vi "TCP Server Module(Multi-Loop Support).vi"(7 "Name (\"\" to Use UUID)":string="Event CSM Tiny") -> ()   [LabVIEW 2017, in "Multi-Loop Module Example.lvlib"]
doc: "------------- lvcsm -------------\n[CSMStates]\nItem 0 = \"Event Structure\"\nItem 1 = \"Idle\"\nItem 2 = \"CSM Documentation\"\nItem 3 = \"VI Reference\"\nItem 4 = \"Error Handler\"\nItem 5 = \"Critical Error\"\nItem 6 = \"Target Error\"\nItem 7 = \"Target Timeout Error\"\nItem 8 = \"Async Response\"\nItem 9 = \"Response\"\nItem 10 = \"Async Message Posted\"\nItem 11 = \"Initialize Core Data\"\nItem 12 = \"Exit\"\nItem 13 = \"Data: Initialize\"\nItem 14 = \"Data: Cleanup\"\nItem 15 = \"Events: Register\"\nItem 16 = \"Events: Unregister\"\nItem 17 = \"UI: Initialize\"\nItem 18 = \"UI: Cursor Set\"\nItem 19 = \"UI: Front Panel State\"\nItem 20 = \"Macro: Initialize\"\nItem 21 = \"Macro: Exit\"\nItem 22 = \"TCP: Send\"\nItem 23 = \"TCP: Receive\"\n\n[CSMStatus]\nItem 0 = \"Error Occurred@Error Handler\"\nItem 1 = \"TCP Received@TCP: Receive\"\nItem 2 = \"TCP Disconnected@\"\nItem 3 = \"TCP Connected@\""
uses:
  Multi-Loop Module Example.lvlib
  user.lib/_NEVSTOP/Communicable State Machine(CSM)/AdvanceAPI/CSM - Make String Arguments Safe.vi
  user.lib/_NEVSTOP/Communicable State Machine(CSM)/AdvanceAPI/CSM - Break Down Multiple States String.vi
  user.lib/_NEVSTOP/Communicable State Machine(CSM)/AdvanceAPI/CSM - Compact Multiple States.vi
  user.lib/_NEVSTOP/Communicable State Machine(CSM)/AdvanceAPI/CSM - Keywords.vi
  user.lib/_NEVSTOP/Communicable State Machine(CSM)/AdvanceAPI/CSM - List Modules.vi
  user.lib/_NEVSTOP/Communicable State Machine(CSM)/Communicable State Machine.lvlib
panel:
  in  "Send String":string
  out "Connected":bool
  out "TCP Received":string
  out "TCP":refnum<k5>
  out "State History":string
  # "#CSM-Example Overview"
  # "#CSM-Example Instructions"
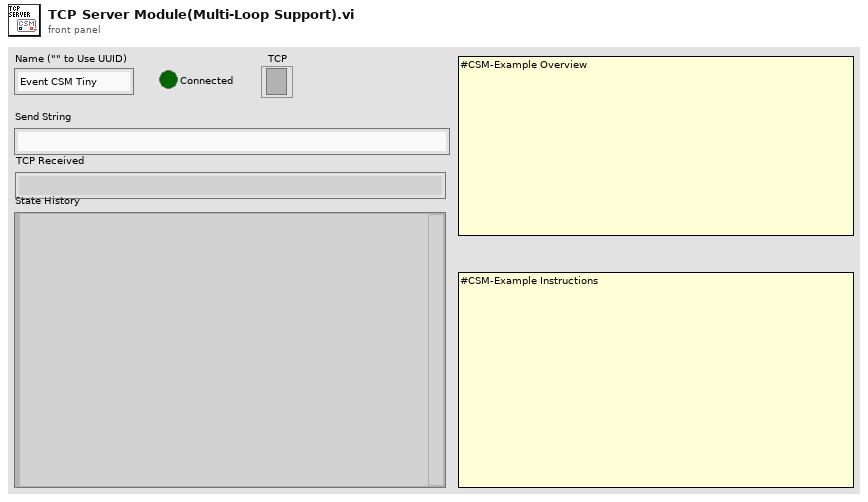
[diagram p1: front panel]
types:
  T1 = enum32{"Invalid", "Standard", "Closed", "Hidden", "Minimized", "Maximized"}
  T2 = enum32{"invalid app kind", "Development System", "Run Time System", "Student Edition", "Embedded LabVIEW", "Evaluation", "Custom"}
  T3 = typedef "Communicable State Machine.lvlib/_CSM_Response Source Message.ctl" = cluster{"‘State":string, "’Arguments":string, "’Error":errorcluster}
  T4 = cluster{"Current VI Reference":refnum<vi>, "Close Panel on Exit?":bool}
  T5 = cluster{"Core":cluster{"Current VI Reference":refnum<vi>, "Close Panel on Exit?":bool}, "Your Boolean data":bool, "Your string data":string}
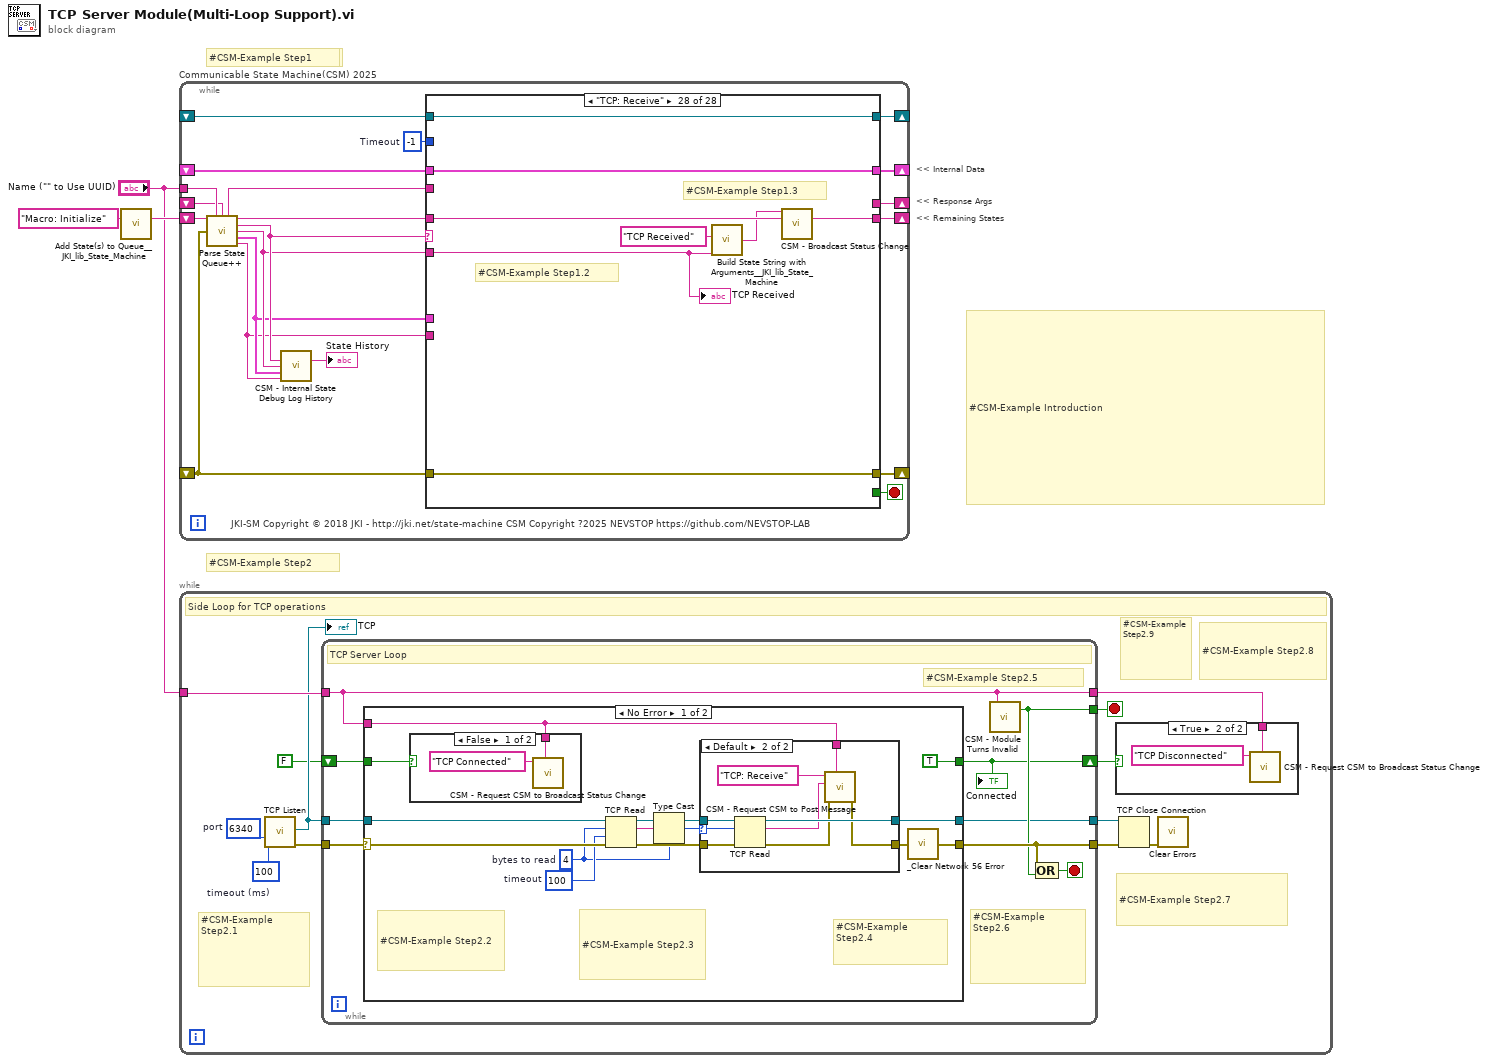
[diagram p0: block diagram]
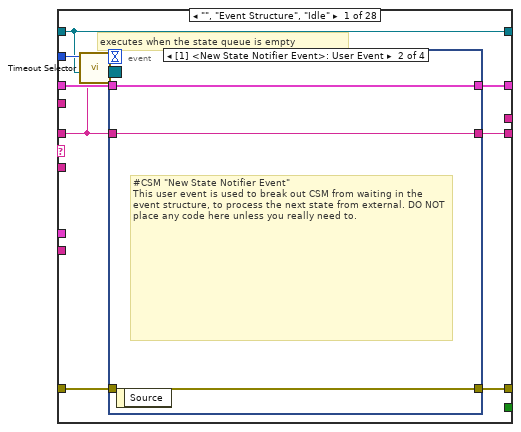
[diagram p2: hidden frame]
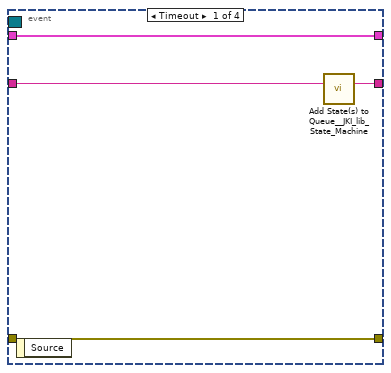
[diagram p3: hidden frame]
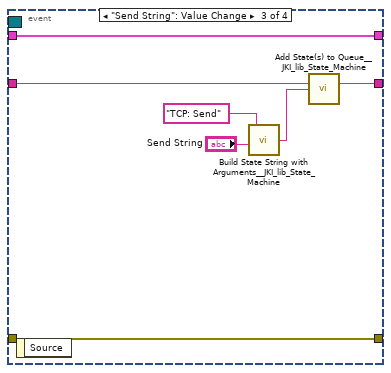
[diagram p4: hidden frame]
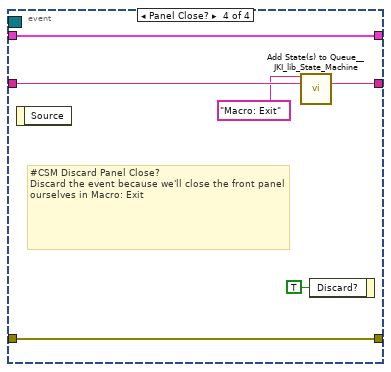
[diagram p5: hidden frame]
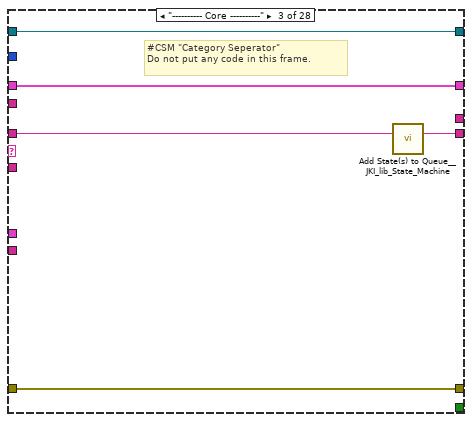
[diagram p7: hidden frame]
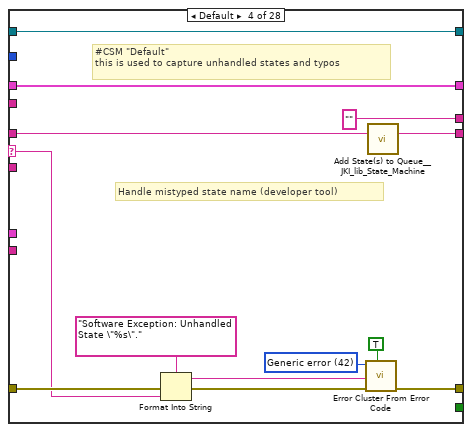
[diagram p8: hidden frame]
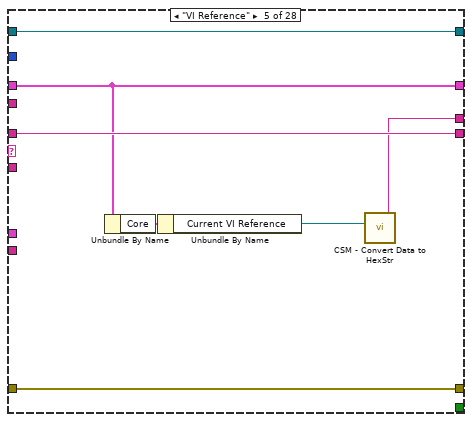
[diagram p9: hidden frame]
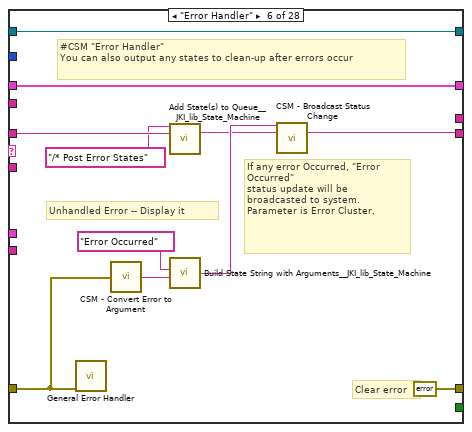
[diagram p10: hidden frame]
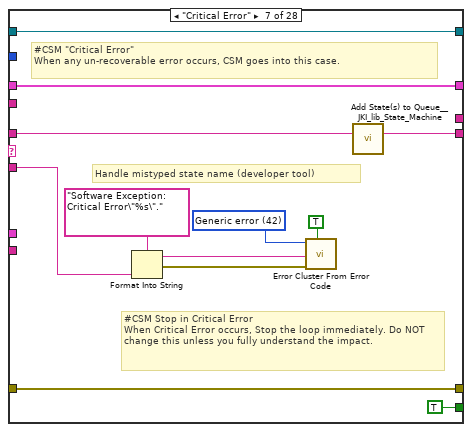
[diagram p11: hidden frame]
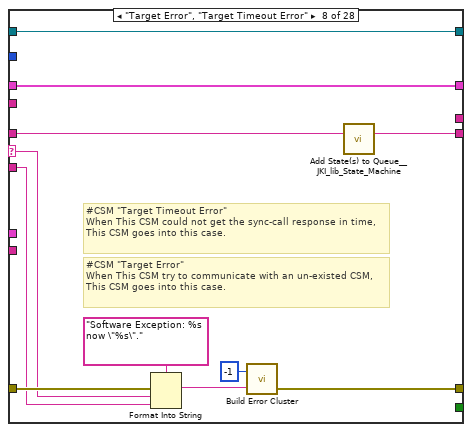
[diagram p12: hidden frame]
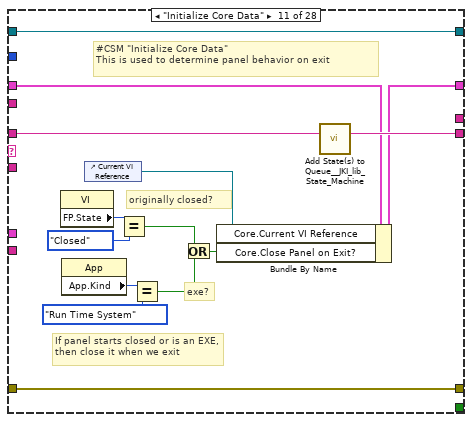
[diagram p15: hidden frame]
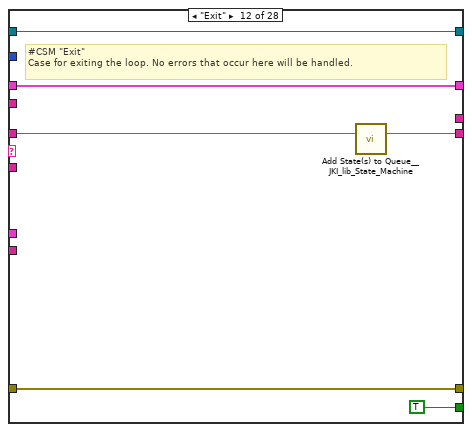
[diagram p16: hidden frame]
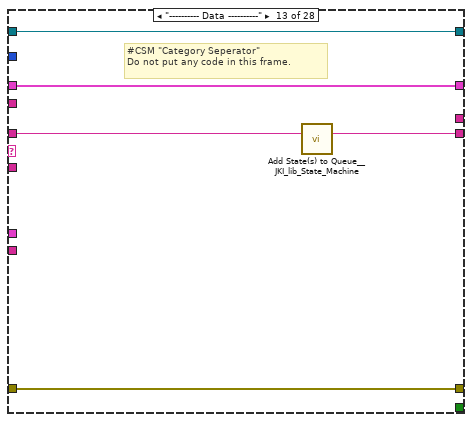
[diagram p17: hidden frame]
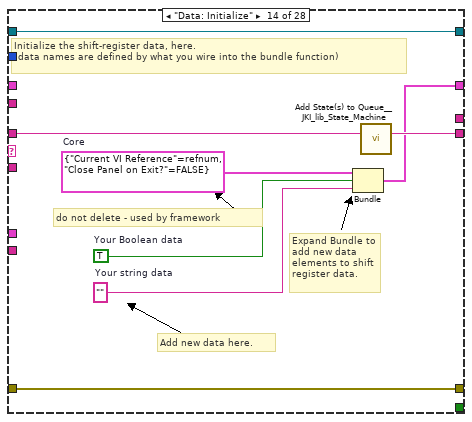
[diagram p18: hidden frame]
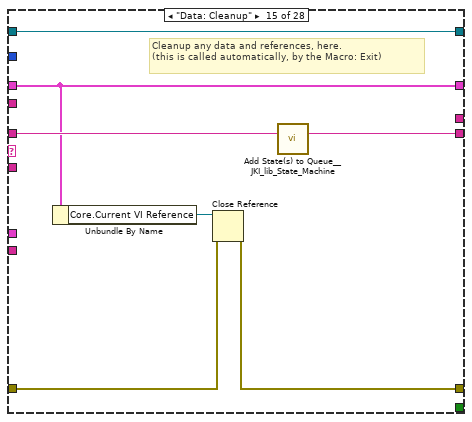
[diagram p19: hidden frame]
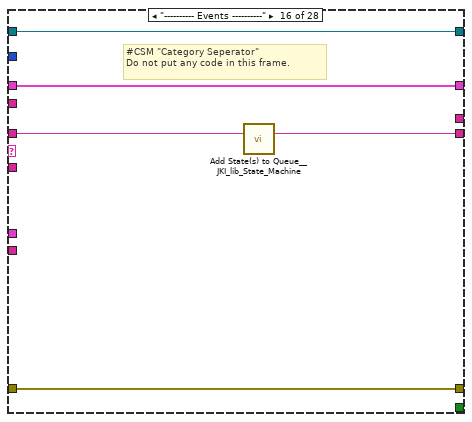
[diagram p20: hidden frame]
diagram:
  # "#CSM-Example Step1"
  # "#CSM-Example Step2"
  # "#CSM-Example Step1"
  # "#CSM-Example Introduction"
  # "<< Internal Data"
  # "<< Response Args"
  # "<< Remaining States"
  n1 = call <vilib>:"Add State(s) to Queue__JKI_lib_State_Machine.vi"("State(s) in (\"\")"="Macro: Initialize") -> ("States Out"=w2:string)  [unwired: 14 in]
  n2 = while "Communicable State Machine(CSM) 2025" {
    shift-right: [w18] -> _
    shift-left: _ -> [w17]
    shift-right: [w21] -> _
    shift-left: _ -> [w15]
    shift-right: [w20] -> _
    shift-left: w2 -> [w22]
    tunnel: "Name (\"\" to Use UUID)" -> [w11]
    shift-right: [w14] -> _
    shift-left: _ -> [w5]
    shift-right: [w13] -> _
    shift-left: _ -> [w12]
    stop <- w19 stop-if-true
    w16 = -1  # Timeout
    # "JKI-SM Copyright © 2018 JKI - http://jki.net/state-machine CSM Copyright ?2025 NEVSTOP https://github.com/NEVSTOP-LAB"
    n3 = call "Parse State Queue++.vi"("State Queue"=w22, "Name (\"\" to Use UUID)"=w11, "Response Arguments"=w5, "Previous Error"=w15) -> ("Name Used"=w6:string, "Remaining States"=w23:string, "Current State"=w10:string, "Arguments"=w9:string, "Additional Information"=w8:T3, "Source CSM"=w7:string)  [unwired: 6 in]
    n4 = call "CSM - Internal State Debug Log History.vi"("State"=w10, "Arguments (\"\")"=w9, ">> Response Source Message >>"=w8, "Source (\"\")"=w7) -> ("Debug Log"=→"State History":string)  [unwired: 11 in]
    n5 = case shown="\"TCP: Receive\"" w10 {
      selector: w10 -> [_ _ _ w64 _ _ _ w108 _ _ _ _ _ _ _ _ _ _ _ _ _ _ _ _ _ _ _ _]
      tunnel: w23 -> [w24 w55 w61 w68 w80 w92 w102 w110 w118 w122 w137 w143 w148 w156 w163 w168 w175 w179 w185 w190 w197 w213 w283 w289 w300 w303 w314 w321]
      tunnel: w9 -> [_ _ _ _ _ _ w95 w109 _ _ _ _ _ _ _ _ _ _ _ _ w192 w207 _ _ _ _ w305 w316]
      tunnel: w17 -> [w31 w54 w58 w66 w79 w90 w103 w112 w117 w121 w130 w141 w145 _ w158 w165 w174 w178 w182 w188 w195 w209 w280 w286 w297 w302 w313 w320]
      tunnel: [w30 w56 w59 w70 w81 errorcluster {"status"=FALSE, "code"=0, "source"=""} ("error out") w104 w106 w119 w123 w134 w140 w146 w153 w159 w166 w169 w177 w183 w187 w193 w210 w281 w287 w298 w304 w306 w322] -> w21
      tunnel: w15 -> [w29 w56 w59 w69 w81 w82 w104 w114 w119 w123 w134 w140 w146 w153 w160 w166 _ w180 w183 w187 w194 w211 w281 w287 w298 w304 _ w322]
      tunnel: [w32 w55 w60 w67 w80 w83 w101 w113 w118 w122 w136 w142 w147 w155 w162 w167 w175 w179 w184 w189 w196 w212 w282 w288 w299 w303 w314 w318] -> w20
      tunnel: [_ _ _ _ _ _ TRUE _ _ _ _ TRUE _ _ _ _ _ _ _ _ _ _ _ _ _ _ _ _] -> w19
      tunnel: [w28 w54 w58 w66 w79 w90 w103 w112 w117 w121 w135 w141 w145 w154 w158 w165 w174 w178 w182 w188 w195 w209 w280 w286 w297 w302 w313 w320] -> w18
      tunnel: w16 -> [w27 _ _ _ _ _ _ _ _ _ _ _ _ _ _ _ _ _ _ _ _ _ _ _ _ _ _ _]
      tunnel: w7 -> [_ _ _ _ _ _ _ _ _ _ _ _ _ _ _ _ _ _ _ _ _ _ _ _ _ _ _ _]
      tunnel: w8 -> [_ _ _ _ _ _ _ _ _ _ _ _ _ _ _ _ _ _ _ _ _ _ _ _ _ _ _ _]
      tunnel: [_ _ _ "" w75 _ _ _ _ _ _ _ _ _ _ _ _ _ _ _ _ _ _ _ _ _ _ _] -> w14
      tunnel: [w26 w53 w57 w62 w78 w88 w93 w111 w116 w120 w124 w138 w144 w149 w157 w164 w173 w176 w181 w186 w191 w206 w279 w284 w290 w301 w312 w319] -> w13
      tunnel: w12 -> [w26 w53 w57 w62 w78 w88 w93 w111 w116 w120 w124 w138 w144 w149 w157 w164 _ w176 w181 w186 w191 w206 w279 w284 w290 w301 w312 w319]
      tunnel: w6 -> [_ _ _ _ _ _ _ _ _ _ _ _ _ _ _ _ w172 _ _ _ _ _ _ _ _ _ _ _]
      frame "", "Event Structure", "Idle" {
        # "executes when the state queue is empty"
        n6 = call "Timeout Selector.vi"("Remaining States"=w24, "Timeout Expected"=w27) -> ("Timeout"=w25:i32)  [unwired: 5 in]
        n7 = event shown="[1] <New State Notifier Event>: User Event" {
          selector: w26 -> [_ _ _ _]
          dyn-events: _ -> [_ _ _ _]
          timeout: w25 -> [_ _ _ _]
          tunnel: w24 -> [w36 w38 w44 w52]
          tunnel: [w35 w38 w43 w51] -> w32
          tunnel: w31 -> [w33 w39 w45 w49]
          tunnel: [w34 w37 w46 w50] -> w30
          tunnel: w29 -> [w34 w37 w46 w50]
          tunnel: [w33 w39 w45 w49] -> w28
          event Timeout {
            n8 = event-data() -> ()  [unwired: 1 in, 1 out]
            n9 = call <vilib>:"Add State(s) to Queue__JKI_lib_State_Machine.vi"("State(s) in (\"\")"=w36) -> ("States Out"=w35:string)  [unwired: 14 in]
          }
          event User Event {
            # "#CSM \"New State Notifier Event\"\nThis user event is used to break out CSM from waiting in the event structure, to process the next state from external. DO NOT place any code here unless you really need to."
            n10 = event-data() -> ()  [unwired: 1 in, 1 out]
          }
          event "Send String": Value Change {
            n11 = event-data() -> ()  [unwired: 1 in, 1 out]
            n12 = call <vilib>:"Build State String with Arguments__JKI_lib_State_Machine.vi"("Arguments (\"\")"="Send String", "State"="TCP: Send") -> ("State with Arguments"=w41:string)  [unwired: 4 in]
            n13 = call <vilib>:"Add State(s) to Queue__JKI_lib_State_Machine.vi"("State(s) in (\"\")"=w44, "State(s) at Back (\"\")"=w41) -> ("States Out"=w43:string)  [unwired: 13 in]
          }
          event Panel Close? {
            # "#CSM Discard Panel Close?\nDiscard the event because we'll close the front panel ourselves in Macro: Exit"
            n14 = event-data() -> ()  [unwired: 1 in, 1 out]
            n15 = call <vilib>:"Add State(s) to Queue__JKI_lib_State_Machine.vi"("State(s) in Front (\"\")"="Macro: Exit", "State(s) in (\"\")"=w52) -> ("States Out"=w51:string)  [unwired: 13 in]
            n16 = event-data("Discard?"=TRUE) -> ()  [unwired: 1 in, 1 out]
          }
        }
      }
      frame "CSM Documentation" {
        # "#CSM README FIRST\n\nCSM is a LabVIEW application framework that builds upon JKI State Machine (JKISM). It follows the pattern of JKISM and extends the keywords to describe message communication between CSM modules, including concepts such as Sync-Message, Async-Message, Subscription/Unsubscription of status - essential elements for creating reusable code modules. For more information, please visit the CSM wiki: https://github.com/NEVSTOP-LAB/JKI-State-Machine-Plus-Plus/wiki\n\nFor instructions on JKI State Machine, visit: http://jki.net/state-machine/\nFor information about CSM, visit: https://github.com/NEVSTOP-LAB"
        # "#CSM \"Documentation\"\nCase for holding CSM Documenation"
      }
      frame "---------- Core ----------" {
        # "#CSM \"Category Seperator\"\nDo not put any code in this frame."
        n17 = call <vilib>:"Add State(s) to Queue__JKI_lib_State_Machine.vi"("State(s) in (\"\")"=w61) -> ("States Out"=w60:string)  [unwired: 14 in]
      }
      frame Default {
        w73 = 42 items=["No error", "Argument error", "Memory is full", "Out of zone", "End of file", "File already open", "Generic file I/O error", "File not found", "File permission error", "Disk is full", "Duplicate path", "Too many files open", "System feature not enabled", "Resource file not found", "Cannot add resource", "Resource not found", "Image not found", "Image memory error", "Pen does not exist", "Config type invalid", "Config token not found", "Config parse error", "Config memory error", "Bad external code format", "Bad external code offset", "External code not present", "Null window", "Destroy window error", "Null menu", "Print aborted", "Bad print record", "Print driver error", "Windows error during printing", "Memory error during printing", "Print dialog error", "Generic print error", "Invalid device refnum", "Device not found", "Device parameter error", "Device unit error", "Cannot open device", "Device call aborted", "Generic error", "Cancelled by user", "Object ID too low", "Object ID too high", "Object not in heap", "Unknown heap", "Unknown object (invalid DefProc)", "Unknown object (DefProc not in table)", "Message out of range", "Invalid (null) method", "Unknown message", "Manager call not supported", "Bad address", "Network operation in progress", "Network operation timed out", "Connection is busy", "Network attribute not supported", "Network error", "Address in use", "System out of memory", "Connection aborted", "Connection refused", "Not connected", "Already connected", "Connection closed", "Initialization error (interapplication manager)", "Bad occurrence", "Wait on unbound occurrence handler", "Occurrence queue overflow", "Datalog type conflict", "Unused", "Unrecognized type (interapplication manager)", "Memory corrupt", "Failed to make temporary DLL", "Old CIN version", "Drag socket not found", "Failed to load drop-object", "Failed to register OLE object", "Failed to release OLE object", "Format specifier type mismatch", "Unknown format specifier", "Too few format specifiers", "Too many format specifiers", "Scan failed", "Newer CIN version", "Error converting to variant", "Runtime menu error", "Password tampered", "Variant attribute not found", "Incompatible variant data type", "Event data is not available", "Event Store is not present", "Occurrence is not found", "Event Queue is not created", "Event info is not available", "Refnum passed is NULL", "Error retrieving Class GUID", "Error retrieving CoClass GUID", "Error retrieving TypeLib GUID.", "Bad built application magic bytes.", "Specific driver is different from the specific driver associated with the Logical Name.", "There is no session opened to the class driver.", "Max Error", "MAX - Error with config objects", "MAX - Error loading configuration", "MAX - Group not supported"]
        # "#CSM \"Default\"\nthis is used to capture unhandled states and typos"
        # "Handle mistyped state name (developer tool)"
        n18 = Format Into String(format string="Software Exception: Unhandled State \"%s\"." ("message"), error in=w69, w64) -> (resulting string=w72:string, error out=w71:errorcluster)  [unwired: 1 in]
        n19 = call <vilib>:"Error Cluster From Error Code.vi"("show call chain? (False)"=TRUE, "error in (no error)"=w71, "error message (\"\")"=w72, "error code (0)"=w73) -> ("error out"=w70:errorcluster)  [unwired: 5 in]
        n20 = call <vilib>:"Add State(s) to Queue__JKI_lib_State_Machine.vi"("State(s) in (\"\")"=w68) -> ("States Out"=w67:string)  [unwired: 14 in]
      }
      frame "VI Reference" {
        n21 = Unbundle By Name(w79) -> ("Core"=w77:T4)
        n22 = Unbundle By Name(w77) -> ("Current VI Reference"=w76:refnum<vi>)
        n23 = call "CSM - Convert Data to HexStr.vi"("Variant"=w76) -> ("HEX String (0-9,A-F)"=w75:string)  [unwired: 8 in]
      }
      frame "Error Handler" {
        # "#CSM \"Error Handler\"\nYou can also output any states to clean-up after errors occur"
        # "If any error Occurred, \"Error Occurred\" \nstatus update will be broadcasted to system.\nParameter is Error Cluster."
        # "Unhandled Error -- Display it"
        # "Clear error"
        n24 = call <vilib>:"General Error Handler.vi"("error in (no error)"=w82) -> ()  [unwired: 10 in, 5 out]
        n25 = call "CSM - Convert Error to Argument.vi"("Error"=w82) -> ("Argument"=w86:string)  [unwired: 4 in]
        n26 = call <vilib>:"Add State(s) to Queue__JKI_lib_State_Machine.vi"("State(s) in Front (\"\")"="/* Post Error States", "State(s) in (\"\")"=w92) -> ("States Out"=w84:string)  [unwired: 13 in]
        n27 = call <vilib>:"Build State String with Arguments__JKI_lib_State_Machine.vi"("Arguments (\"\")"=w86, "State"="Error Occurred" ("Status with Arguments")) -> ("State with Arguments"=w85:string)  [unwired: 4 in]
        n28 = call "CSM - Broadcast Status Change.vi"("Status With Arguments"=w85, "State Queue"=w84) -> ("Remaining States"=w83:string)  [unwired: 13 in]
      }
      frame "Critical Error" {
        w99 = 42 items=["No error", "Argument error", "Memory is full", "Out of zone", "End of file", "File already open", "Generic file I/O error", "File not found", "File permission error", "Disk is full", "Duplicate path", "Too many files open", "System feature not enabled", "Resource file not found", "Cannot add resource", "Resource not found", "Image not found", "Image memory error", "Pen does not exist", "Config type invalid", "Config token not found", "Config parse error", "Config memory error", "Bad external code format", "Bad external code offset", "External code not present", "Null window", "Destroy window error", "Null menu", "Print aborted", "Bad print record", "Print driver error", "Windows error during printing", "Memory error during printing", "Print dialog error", "Generic print error", "Invalid device refnum", "Device not found", "Device parameter error", "Device unit error", "Cannot open device", "Device call aborted", "Generic error", "Cancelled by user", "Object ID too low", "Object ID too high", "Object not in heap", "Unknown heap", "Unknown object (invalid DefProc)", "Unknown object (DefProc not in table)", "Message out of range", "Invalid (null) method", "Unknown message", "Manager call not supported", "Bad address", "Network operation in progress", "Network operation timed out", "Connection is busy", "Network attribute not supported", "Network error", "Address in use", "System out of memory", "Connection aborted", "Connection refused", "Not connected", "Already connected", "Connection closed", "Initialization error (interapplication manager)", "Bad occurrence", "Wait on unbound occurrence handler", "Occurrence queue overflow", "Datalog type conflict", "Unused", "Unrecognized type (interapplication manager)", "Memory corrupt", "Failed to make temporary DLL", "Old CIN version", "Drag socket not found", "Failed to load drop-object", "Failed to register OLE object", "Failed to release OLE object", "Format specifier type mismatch", "Unknown format specifier", "Too few format specifiers", "Too many format specifiers", "Scan failed", "Newer CIN version", "Error converting to variant", "Runtime menu error", "Password tampered", "Variant attribute not found", "Incompatible variant data type", "Event data is not available", "Event Store is not present", "Occurrence is not found", "Event Queue is not created", "Event info is not available", "Refnum passed is NULL", "Error retrieving Class GUID", "Error retrieving CoClass GUID", "Error retrieving TypeLib GUID.", "Bad built application magic bytes.", "Specific driver is different from the specific driver associated with the Logical Name.", "There is no session opened to the class driver.", "Max Error", "MAX - Error with config objects", "MAX - Error loading configuration", "MAX - Group not supported"]
        # "#CSM Stop in Critical Error\nWhen Critical Error occurs, Stop the loop immediately. Do NOT change this unless you fully understand the impact."
        # "#CSM \"Critical Error\"\nWhen any un-recoverable error occurs, CSM goes into this case."
        # "Handle mistyped state name (developer tool)"
        n29 = Format Into String(format string="Software Exception: Critical Error\"%s\"." ("message"), w95) -> (resulting string=w98:string, error out=w97:errorcluster)  [unwired: 2 in]
        n30 = call <vilib>:"Error Cluster From Error Code.vi"("show call chain? (False)"=TRUE, "error in (no error)"=w97, "error message (\"\")"=w98, "error code (0)"=w99) -> ()  [unwired: 5 in, 1 out]
        n31 = call <vilib>:"Add State(s) to Queue__JKI_lib_State_Machine.vi"("State(s) in (\"\")"=w102) -> ("States Out"=w101:string)  [unwired: 14 in]
      }
      frame "Target Error", "Target Timeout Error" {
        # "#CSM \"Target Error\"\nWhen This CSM try to communicate with an un-existed CSM, This CSM goes into this case."
        # "#CSM \"Target Timeout Error\"\nWhen This CSM could not get the sync-call response in time, This CSM goes into this case."
        n32 = Format Into String(format string="Software Exception: %s now \"%s\"." ("message"), error in=w114, w108, w109) -> (resulting string=w107:string)  [unwired: 1 in, 1 out]
        n33 = call "Build Error Cluster.vi"("String to Prepend to Source (\"\")"=w107, "Code"=-1 ("code")) -> ("error out"=w106:errorcluster)
        n34 = call <vilib>:"Add State(s) to Queue__JKI_lib_State_Machine.vi"("State(s) in (\"\")"=w110) -> ("States Out"=w113:string)  [unwired: 14 in]
      }
      frame "Async Response", "Response" {
        # "#CSM Response Comments\nAfter Message is executed, CSM goes to this state for receive the response.\n    For Async Message(->), \"Async Response\" is used. This CSM will goes to \"Async Message Posted\" immediately and receive the \"Async Response\" after the callee finishes the message.\n    For Sync Message(@),  This CSM will wait until the message is done and immediately goes to \"Response\""
        # "#CSM \"Async Response\"\nHandle Async-call Response (\"Async Response\" for ->)"
        # "#CSM \"Response\"\nHandle Sync-call Response (\"Response\" for -@)"
      }
      frame "Async Message Posted" {
        # "#CSM \"Async Message Posted\"\nAfter Async Message is posted (-> or ->| ), CSM goes to this state for post-action.\nYou can use Argument - State to tell which Async Message is called."
      }
      frame "Initialize Core Data" {
        # "#CSM \"Initialize Core Data\"\nThis is used to determine panel behavior on exit"
        # "originally closed?"
        # "exe?"
        # "If panel starts closed or is an EXE, then close it when we exit"
        n35 = property class="VI"() -> ("FP.State"=w127:T1)  [unwired: 2 in, 2 out]
        n36 = property class="App"() -> ("App.Kind"=w133:T2)  [unwired: 2 in, 2 out]
        n37 = control-ref of="Current VI Reference"() -> (w128:refnum<vi>)
        n38 = Equal?(x=w127, y=T1."Closed" ("Front Panel Window:State")) -> (x = y?=w125:bool)
        n39 = Equal?(x=w133, y=T2."Run Time System" ("Application:Kind")) -> (x = y?=w131:bool)
        n40 = Or(x=w125, y=w131) -> (x .or. y?=w129:bool)
        n41 = Bundle By Name(cluster=w130, "Core.Current VI Reference"=w128, "Core.Close Panel on Exit?"=w129) -> (w135:T5)
        n42 = call <vilib>:"Add State(s) to Queue__JKI_lib_State_Machine.vi"("State(s) in (\"\")"=w137) -> ("States Out"=w136:string)  [unwired: 14 in]
      }
      frame "Exit" {
        # "#CSM \"Exit\"\nCase for exiting the loop. No errors that occur here will be handled."
        n43 = call <vilib>:"Add State(s) to Queue__JKI_lib_State_Machine.vi"("State(s) in (\"\")"=w143) -> ("States Out"=w142:string)  [unwired: 14 in]
      }
      frame "---------- Data ----------" {
        # "#CSM \"Category Seperator\"\nDo not put any code in this frame."
        n44 = call <vilib>:"Add State(s) to Queue__JKI_lib_State_Machine.vi"("State(s) in (\"\")"=w148) -> ("States Out"=w147:string)  [unwired: 14 in]
      }
      frame "Data: Initialize" {
        w150 = T4 {"Current VI Reference"=refnum, "Close Panel on Exit?"=FALSE}  # Core
        w152 = TRUE  # Your Boolean data
        w151 = ""  # Your string data
        # "do not delete - used by framework"
        # "Expand Bundle to add new data elements to shift register data."
        # "Add new data here."
        # "Initialize the shift-register data, here.\n(data names are defined by what you wire into the bundle function)"
        n45 = Bundle("Core"=w150, "Your Boolean data"=w152, "Your string data"=w151) -> (w154:T5)  [unwired: 1 in]
        n46 = call <vilib>:"Add State(s) to Queue__JKI_lib_State_Machine.vi"("State(s) in (\"\")"=w156) -> ("States Out"=w155:string)  [unwired: 14 in]
      }
      frame "Data: Cleanup" {
        # "Cleanup any data and references, here.\n(this is called automatically, by the Macro: Exit)"
        n47 = Unbundle By Name(w158) -> ("Core.Current VI Reference"=w161:refnum<vi>)
        n48 = Close Reference(reference=w161, error in (no error)=w160) -> (error out=w159:errorcluster)
        n49 = call <vilib>:"Add State(s) to Queue__JKI_lib_State_Machine.vi"("State(s) in (\"\")"=w163) -> ("States Out"=w162:string)  [unwired: 14 in]
      }
      frame "---------- Events ----------" {
        # "#CSM \"Category Seperator\"\nDo not put any code in this frame."
        n50 = call <vilib>:"Add State(s) to Queue__JKI_lib_State_Machine.vi"("State(s) in (\"\")"=w168) -> ("States Out"=w167:string)  [unwired: 14 in]
      }
      frame "Events: Register" {
        # "#CSM \"Events: Register\"\nRegister user event. New Message Event is registered to break CSM waiting in event structure by default."
        # "#CSM Register New Message Event\nRegister message event to break Waiting in Event structure."
        n51 = call "CSM - Get New State Notifier Event.vi"("Name (\"\" to Use UUID)"=w172) -> ("error out"=w170:errorcluster, "New State Notifier Event"=w171:refnum<user-event>)  [unwired: 9 in]
        n52 = register-events(error in=w170, w171) -> (reference out=w173:refnum<event-registration>, error out=w169:errorcluster)  [unwired: 1 in]
      }
      frame "Events: Unregister" {
        # "#CSM \"Events: Unregister\"\nUnregister user event."
        n53 = Unregister For Events(event registration refnum=w176, error in=w180) -> (error out=w177:errorcluster)
      }
      frame "---------- UI ----------" {
        # "#CSM \"Category Seperator\"\nDo not put any code in this frame."
        n54 = call <vilib>:"Add State(s) to Queue__JKI_lib_State_Machine.vi"("State(s) in (\"\")"=w185) -> ("States Out"=w184:string)  [unwired: 14 in]
      }
      frame "UI: Initialize" {
        # "#CSM \"UI: Initialize\"\nInitialize the User Interface, here.\n(this is called automatically, by the Macro: Init)"
        n55 = call <vilib>:"Add State(s) to Queue__JKI_lib_State_Machine.vi"("State(s) in (\"\")"=w190) -> ("States Out"=w189:string)  [unwired: 14 in]
      }
      frame "UI: Cursor Set" {
        # "#CSM \"UI: Cursor Set\"\nSet and Unset Cursor Busy.\n(Usage: \"UI: Cursor Set >> Busy|Idle\")"
        # "Argument"
        n56 = disable-structure shown="TARGET_TYPE!=Windows" {
          disable-tunnel: w194 -> [w200 w205]
          disable-tunnel: [w199 w205] -> w193
          disable-tunnel: w192 -> [w198 _]
          frame condition #0 (active) {
            n57 = case shown="\"Idle\", Default" w198 {
              tunnel: w200 -> [w202 w204]
              tunnel: [w201 w203] -> w199
              frame "Idle", Default {
                n58 = call <vilib>:"Unset Busy.vi"("error in (no error)"=w202) -> ("error out"=w201:errorcluster)  [unwired: 10 in]
              }
              frame "Busy" {
                n59 = call <vilib>:"Set Busy.vi"("error in (no error)"=w204) -> ("error out"=w203:errorcluster)  [unwired: 9 in, 1 out]
              }
            }
          }
          frame condition #1 {
          }
        }
        n60 = call <vilib>:"Add State(s) to Queue__JKI_lib_State_Machine.vi"("State(s) in (\"\")"=w197) -> ("States Out"=w196:string)  [unwired: 14 in]
      }
      frame "UI: Front Panel State" {
        # "#CSM \"UI: Front Panel State\"\nSet Front Panel Open or Closed\n(Usage: \"UI: Front Panel State >> Open|Close\")"
        # "Argument"
        n61 = Unbundle By Name(w209) -> ("Core.Current VI Reference"=w208:refnum<vi>)
        n62 = call <vilib>:"Add State(s) to Queue__JKI_lib_State_Machine.vi"("State(s) in (\"\")"=w213) -> ("States Out"=w212:string)  [unwired: 14 in]
        n63 = case shown="\"Close\", \"Closed\"" w207 {
          tunnel: w211 -> [w219 w234 w245 w258 w271]
          tunnel: [w221 w235 w247 w260 w273] -> w210
          tunnel: w208 -> [w220 w232 w246 w259 w272]
          frame "Open", "Standard", Default {
            w214 = T1."Standard" ("State")
            n64 = property class="VI"(reference=w220, error in=w219) -> (reference out=w217:refnum<vi>, error out=w218:errorcluster, "FP.State"=w216:T1)
            n65 = Not Equal?(x=w216, y=w214) -> (x != y?=w215:bool)
            n66 = case shown="True" w215 {
              tunnel: [w225 w227] -> w221
              tunnel: w218 -> [w224 w227]
              tunnel: w217 -> [w223 _]
              tunnel: w214 -> [w222 _]
              frame True {
                n67 = invoke class="VI" method="FP.Open"(reference=w223, error in=w224, "Activate"=TRUE, "State"=w222) -> (error out=w225:errorcluster)  [unwired: 1 in, 4 out]
              }
              frame False {
              }
            }
          }
          frame "Close", "Closed" {
            n68 = property class="VI"(reference=w232, error in=w234) -> (reference out=w231:refnum<vi>, error out=w233:errorcluster, "FP.State"=w229:T1)
            n69 = Not Equal?(x=w229, y=T1."Closed" ("Front Panel Window:State")) -> (x != y?=w228:bool)
            n70 = case shown="False" w228 {
              tunnel: [w236 w239] -> w235
              tunnel: w233 -> [w236 w238]
              tunnel: w231 -> [_ w237]
              frame False {
              }
              frame True {
                n71 = invoke class="VI" method="FP.Close"(reference=w237, error in=w238) -> (error out=w239:errorcluster)  [unwired: 1 in, 2 out]
              }
            }
          }
          frame "Hidden", "Hide" {
            w240 = T1."Hidden" ("State")
            n72 = property class="VI"(reference=w246, error in=w245) -> (reference out=w243:refnum<vi>, error out=w244:errorcluster, "FP.State"=w242:T1)
            n73 = Not Equal?(x=w242, y=w240) -> (x != y?=w241:bool)
            n74 = case shown="True" w241 {
              tunnel: [w251 w252] -> w247
              tunnel: w244 -> [w250 w252]
              tunnel: w243 -> [w249 _]
              tunnel: w240 -> [w248 _]
              frame True {
                n75 = invoke class="VI" method="FP.Open"(reference=w249, error in=w250, "State"=w248) -> (error out=w251:errorcluster)  [unwired: 2 in, 4 out]
              }
              frame False {
              }
            }
          }
          frame "Minimize", "Minimized" {
            w253 = T1."Minimized" ("State")
            n76 = property class="VI"(reference=w259, error in=w258) -> (reference out=w256:refnum<vi>, error out=w257:errorcluster, "FP.State"=w255:T1)
            n77 = Not Equal?(x=w255, y=w253) -> (x != y?=w254:bool)
            n78 = case shown="True" w254 {
              tunnel: [w264 w265] -> w260
              tunnel: w257 -> [w263 w265]
              tunnel: w256 -> [w262 _]
              tunnel: w253 -> [w261 _]
              frame True {
                n79 = invoke class="VI" method="FP.Open"(reference=w262, error in=w263, "State"=w261) -> (error out=w264:errorcluster)  [unwired: 2 in, 4 out]
              }
              frame False {
              }
            }
          }
          frame "Maximize", "Maximized" {
            w266 = T1."Maximized" ("State")
            n80 = property class="VI"(reference=w272, error in=w271) -> (reference out=w269:refnum<vi>, error out=w270:errorcluster, "FP.State"=w268:T1)
            n81 = Not Equal?(x=w268, y=w266) -> (x != y?=w267:bool)
            n82 = case shown="True" w267 {
              tunnel: [w277 w278] -> w273
              tunnel: w270 -> [w276 w278]
              tunnel: w269 -> [w275 _]
              tunnel: w266 -> [w274 _]
              frame True {
                n83 = invoke class="VI" method="FP.Open"(reference=w275, error in=w276, "State"=w274) -> (error out=w277:errorcluster)  [unwired: 2 in, 4 out]
              }
              frame False {
              }
            }
          }
        }
      }
      frame "---------- Macro ----------" {
        # "#CSM \"Category Seperator\"\nDo not put any code in this frame."
        n84 = call <vilib>:"Add State(s) to Queue__JKI_lib_State_Machine.vi"("State(s) in (\"\")"=w283) -> ("States Out"=w282:string)  [unwired: 14 in]
      }
      frame "Macro: Initialize" {
        w285 = "Data: Initialize\nInitialize Core Data\nEvents: Register\nUI: Initialize\n//UI: Front Panel State >> Open"  # Data: Initialize Initialize Core Data Events: Register UI: Initialize //UI: Front Panel State >> Open
        # "#CSM \"Macro: Initialize\"\nInitialization Macro (This is called once, when the VI starts)"
        n85 = call <vilib>:"Add State(s) to Queue__JKI_lib_State_Machine.vi"("State(s) in Front (\"\")"=w285, "State(s) in (\"\")"=w289) -> ("States Out"=w288:string)  [unwired: 13 in]
      }
      frame "Macro: Exit" {
        # "#CSM \"Macro: Exit\"\nExit Macro (This is called once, when the VI exits)"
        n86 = Unbundle By Name(w297) -> ("Core.Close Panel on Exit?"=w296:bool)
        n87 = Select(t="UI: Front Panel State >> Close", s=w296, f="") -> (s? t:f=w293:string)
        n88 = call <vilib>:"Add State(s) to Queue__JKI_lib_State_Machine.vi"("State(s) in (\"\")"=w293, "State(s) at Back (\"\")"="Data: Cleanup\nEvents: Unregister\nExit") -> ("States Out"=w291:string)  [unwired: 13 in]
        n89 = call <vilib>:"Add State(s) to Queue__JKI_lib_State_Machine.vi"("State(s) in Front (\"\")"=w291, "State(s) in (\"\")"=w300) -> ("States Out"=w299:string)  [unwired: 13 in]
      }
      frame "---------- API ----------" {
        # "#CSM \"Category Seperator\"\nDo not put any code in this frame."
      }
      frame "TCP: Send" {
        # "#CSM-Example Step1.1"
        n90 = local read "TCP"() -> (w307:refnum<k5>)
        n91 = String Length(string=w305) -> (length=w309:i32)
        n92 = Type Cast(x=w309) -> (*(type *) &x=w308:string)  [unwired: 1 out]
        n93 = TCP Write(connection ID=w307, data in=w308) -> (connection ID out=w311:refnum<k5>, error out=w310:errorcluster)  [unwired: 1 in, 2 out]
        n94 = TCP Write(connection ID=w311, data in=w305, error in (no error)=w310) -> (error out=w306:errorcluster)  [unwired: 3 out]
      }
      frame "TCP: Receive" {
        # "#CSM-Example Step1.3"
        # "#CSM-Example Step1.2"
        n95 = call <vilib>:"Build State String with Arguments__JKI_lib_State_Machine.vi"("Arguments (\"\")"=w316, "State"="TCP Received") -> ("State with Arguments"=w315:string)  [unwired: 4 in]
        n96 = call "CSM - Broadcast Status Change.vi"("Status With Arguments"=w315, "State Queue"=w321) -> ("Remaining States"=w318:string)  [unwired: 13 in]
        "TCP Received" <- w316
      }
    }
  }
  n97 = while {
    tunnel: "Name (\"\" to Use UUID)" -> [w329]
    stop <- w330 stop-if-true
    w331 = u16 6340  # port
    w332 = 100  # timeout (ms)
    # "#CSM-Example Step2.9"
    # "#CSM-Example Step2.7"
    # "#CSM-Example Step2.8"
    # "#CSM-Example Step2.1"
    # "Side Loop for TCP operations"
    n98 = call <vilib>:"TCP Listen.vi"("timeout ms (wait forever: -1)"=w332, "port"=w331) -> ("error out"=w333:errorcluster, "connection ID"=w328:refnum<k5>)  [unwired: 5 in, 3 out]
    "TCP" <- w328
    n99 = while {
      tunnel: [w344] -> w325
      tunnel: [w340] -> w334
      tunnel: w328 -> [w342]
      tunnel: w333 -> [w341]
      tunnel: [w343] -> w330
      tunnel: w329 -> [w338]
      tunnel: [w338] -> w326
      shift-right: [w337] -> w323
      shift-left: FALSE -> [w339]
      stop <- w345 stop-if-true
      # "#CSM-Example Step2.5"
      # "#CSM-Example Step2.6"
      # "TCP Server Loop"
      n100 = case shown="No Error" w341 {
        selector: w341 -> [w357 w376]
        tunnel: [w359 w376] -> w344
        tunnel: w342 -> [w358 w375]
        tunnel: [w354 w375] -> w340
        tunnel: w339 -> [w348 _]
        tunnel: w338 -> [w349 _]
        tunnel: [TRUE FALSE] -> w337
        frame No Error {
          w351 = 100  # timeout
          w346 = 4  # bytes to read
          # "#CSM-Example Step2.4"
          # "#CSM-Example Step2.3"
          # "#CSM-Example Step2.2"
          n101 = case shown="False" w348 {
            tunnel: w349 -> [w372 _]
            frame False {
              n102 = call "CSM - Request CSM to Broadcast Status Change.vi"("Module Name"=w372, "Status"="TCP Connected") -> ()  [unwired: 9 in, 1 out]
            }
            frame True {
            }
          }
          n103 = TCP Read(connection ID=w358, bytes to read=w346, error in (no error)=w357, 9:w351) -> (connection ID out=w355:refnum<k5>, data out=w353:string, error out=w356:errorcluster)  [unwired: 1 out]
          n104 = Type Cast(type=w346, x=w353) -> (*(type *) &x=w352:i32)
          n105 = case shown="Default" w352 {
            selector: w352 -> [_ w367]
            tunnel: w356 -> [w360 w370]
            tunnel: w355 -> [w361 w369]
            tunnel: [w361 w368] -> w354
            tunnel: [w360 w364] -> w350
            tunnel: w349 -> [_ w363]
            frame 0 {
            }
            frame Default {
              n106 = TCP Read(connection ID=w369, bytes to read=w367, error in (no error)=w370) -> (connection ID out=w368:refnum<k5>, data out=w362:string, error out=w365:errorcluster)  [unwired: 2 out]
              n107 = call "CSM - Request CSM to Post Message.vi"("Module Name"=w363, "Error In (No Error)"=w365, "Arguments (\"\")"=w362, "State"="TCP: Receive") -> ("error out"=w364:errorcluster)  [unwired: 7 in]
            }
          }
          n108 = call "_Clear Network 56 Error.vi"("error in (no error)"=w350) -> ("error out"=w359:errorcluster)  [unwired: 4 in]
        }
        frame Error {
          # "Side-Loop 2. No Connection is created. Wait 100ms for reconnection"
          n109 = Wait (ms)(milliseconds to wait=u32 100) -> ()  [unwired: 1 out]
        }
      }
      "Connected" <- w337
      n110 = call "CSM - Module Turns Invalid.vi"("CSM Name"=w338) -> ("Turn Invalid (Exit)?"=w343:bool)  [unwired: 2 in]
      n111 = Compound Arithmetic op=OR(w344, w343) -> (w345:bool)
    }
    n112 = case shown="True" w323 {
      tunnel: w326 -> [_ w336]
      frame False {
      }
      frame True {
        n113 = call "CSM - Request CSM to Broadcast Status Change.vi"("Module Name"=w336, "Status"="TCP Disconnected") -> ()  [unwired: 9 in, 1 out]
      }
    }
    n114 = TCP Close Connection(connection ID=w334, error in (no error)=w325) -> (error out=w327:errorcluster)  [unwired: 2 out]
    n115 = call <vilib>:"Clear Errors.vi"("error in (no error)"=w327) -> ()  [unwired: 5 in, 2 out]
  }
